vi "ASK_GenPicture.vi"(4 "error in (no error)":errorcluster caption="错误输入（无错误）", 6 "write_filename":string, 7 "N":dbl, 8 "M":dbl, 9 "pic_model":i32, 10 "re_bits":dbl[](array[numeric]), 11 "PathIn":path) -> (0 "error out":errorcluster caption="错误输出", 3 "PathOut":path)   [LabVIEW 2015]
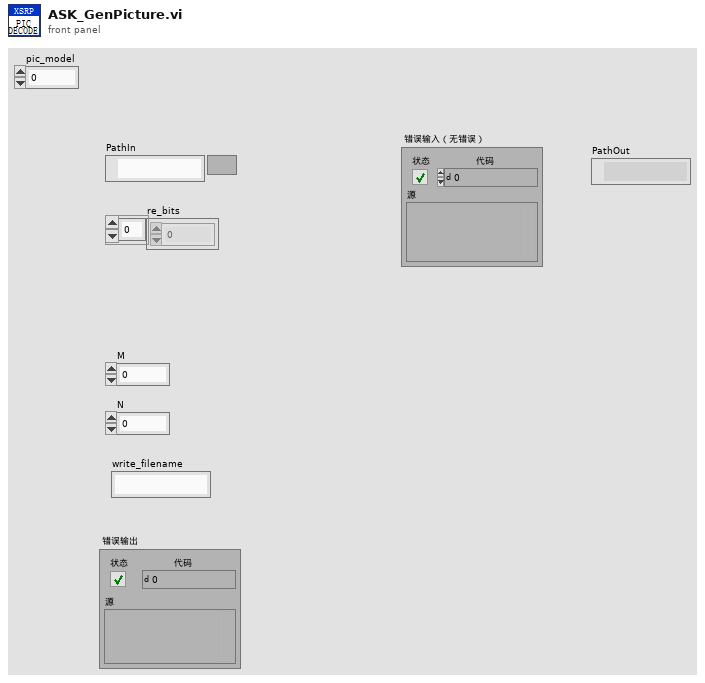
[diagram p1: front panel]
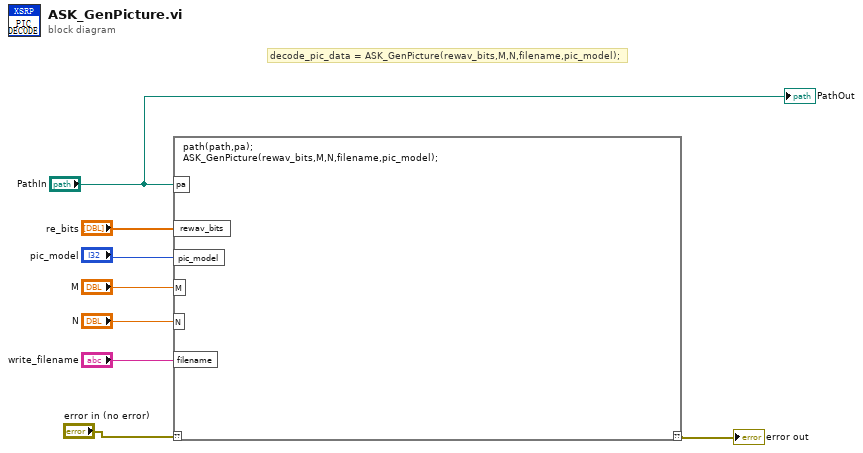
[diagram p0: block diagram]
diagram:
  # "decode_pic_data = ASK_GenPicture(rewav_bits,M,N,filename,pic_model);"
  n1 = script code="path(path,pa);\nASK_GenPicture(rewav_bits,M,N,filename,pic_model);"("??"="error in (no error)", "pa"="PathIn", "M"="M", "N"="N", "rewav_bits"="re_bits", "filename"="write_filename", "pic_model"="pic_model") -> ("??"=→"error out":errorcluster)
  "PathOut" <- "PathIn"
